vi "rotarray.vi"(8 "Pixel Center":cluster{i16, i16}, 9 "Angle":i16, 11 "Array in":cluster{i16, i16}[](array[cluster])) -> (3 "Array out":cluster{dbl, dbl}[](array[cluster]) {"?" format="%.2f"; "?" format="%.2f"})   [LabVIEW 2023]
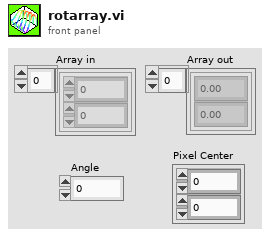
[diagram p1: front panel]
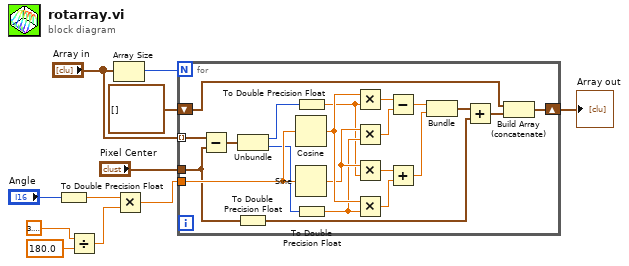
[diagram p0: block diagram]
diagram:
  n1 = To Double Precision Float(number="Angle") -> (double precision float=w1:dbl)
  n2 = Divide(x=3.141592653589793, y=180.0) -> (x/y=w6:dbl)
  n3 = Array Size(array="Array in") -> (size(s)=w9:i32)
  n4 = Multiply(x=w1, y=w6) -> (x*y=w5:dbl)
  n5 = for {
    N: w9 -> [_]
    shift-right: [w32] -> w3
    shift-left: cluster{dbl, dbl}[] [] -> [w31]
    tunnel: w5 -> [w28]
    tunnel: "Array in" -> [w21] mode=indexing
    tunnel: "Pixel Center" -> [w13]
    n6 = Subtract(x=w21, y=w13) -> (x-y=w20:cluster{i16, i16})
    n7 = Unbundle(w20) -> (w17:i16, w16:i16)
    n8 = To Double Precision Float(number=w13) -> (double precision float=w12:cluster{dbl, dbl})
    n9 = Cosine(x=w28) -> (cos(x)=w19:dbl)
    n10 = Sine(x=w28) -> (sin(x)=w18:dbl)
    n11 = To Double Precision Float(number=w17) -> (double precision float=w14:dbl)
    n12 = To Double Precision Float(number=w16) -> (double precision float=w15:dbl)
    n13 = Multiply(x=w19, y=w14) -> (x*y=w25:dbl)
    n14 = Multiply(x=w18, y=w15) -> (x*y=w24:dbl)
    n15 = Multiply(x=w18, y=w14) -> (x*y=w27:dbl)
    n16 = Multiply(x=w19, y=w15) -> (x*y=w26:dbl)
    n17 = Subtract(x=w25, y=w24) -> (x-y=w30:dbl)
    n18 = Add(x=w27, y=w26) -> (x+y=w29:dbl)
    n19 = Bundle(w30, w29) -> (w23:cluster{dbl, dbl})  [unwired: 1 in]
    n20 = Add(x=w23, y=w12) -> (x+y=w22:cluster{dbl, dbl})
    n21 = Build Array (concatenate)(w31, w22) -> (w32:cluster{dbl, dbl}[])
  }
  "Array out" <- w3
